vi "Open.vi"(8 "error in (no error)":errorcluster, 11 "PS Test in":refnum<class "PS Test.lvclass">) -> (0 "error out":errorcluster, 3 "PS Test out":refnum<class "PS Test.lvclass">)   [LabVIEW 2021, in "PS.lvlib" / "PS Test.lvclass"]
uses:
  PS Test.lvclass
  PS/PS.lvclass
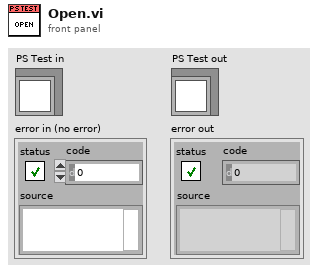
[diagram p1: front panel]
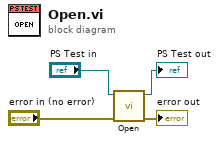
[diagram p0: block diagram]
diagram:
  n1 = call-parent "Open.vi"("error in (no error)"="error in (no error)", "PS in"="PS Test in") -> ("error out"=→"error out":errorcluster, "PS out"=→"PS Test out":refnum<class "PS Test.lvclass">)  [unwired: 8 in]
